vi "Test Billete 100.vi"(8 "error in (no error)":errorcluster, 11 "TestCase in":refnum<class "Unit Test Proy.lvclass">) -> (0 "error out":errorcluster, 3 "TestCase out":refnum<class "Unit Test Proy.lvclass">)   [LabVIEW 2020, in "Unit Test Proy.lvclass"]
uses:
  Unit Test Proy.lvclass
  Dinero/Dinero.lvclass
  Dinero/Dinero.lvclass/Dinero.ctl
  <vilib>/addons/_JKI Toolkits/VI Tester/TestCase.llb/TestCase.lvclass
  C:/Program Files (x86)/National Instruments/LabVIEW 2020/vi.lib/addons/_JKI Toolkits/VI Tester/TestCase.llb/TestCase.lvclass
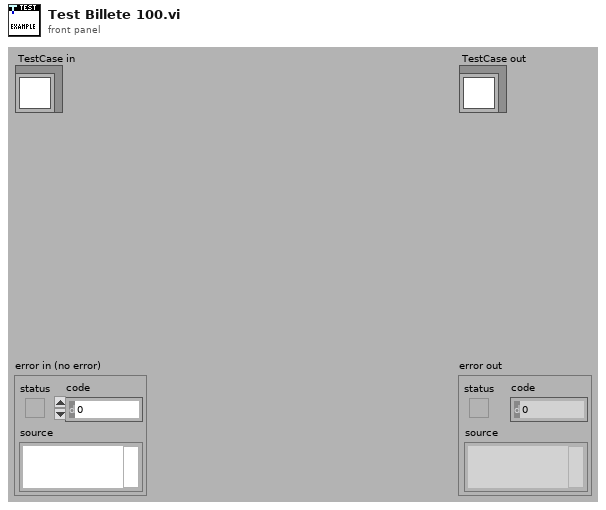
[diagram p1: front panel]
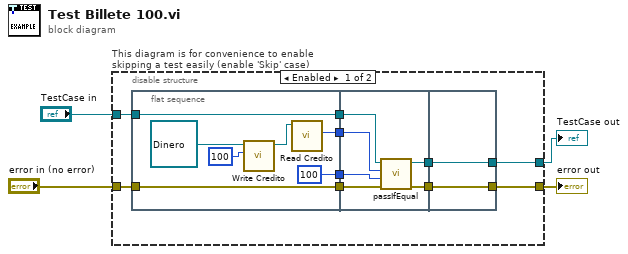
[diagram p0: block diagram]
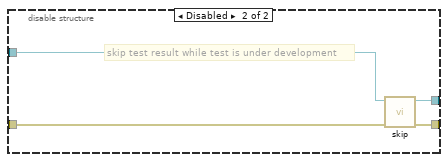
[diagram p2: hidden frame]
diagram:
  n1 = disable-structure "This diagram is for convenience to enable skipping a test easily (enable 'Skip' case)" shown="Enabled" {
    disable-tunnel: "TestCase in" -> [w7 w33]
    disable-tunnel: [w12 w31] -> w1
    disable-tunnel: [w11 w32] -> w3
    disable-tunnel: "error in (no error)" -> [w14 w30]
    frame Enabled {
      n2 = flat-sequence {
        tunnel: w14 -> [w21]
        tunnel: [w21] -> w9
        tunnel: [w20] -> w8
        tunnel: w7 -> [w20]
        tunnel: [w17] -> w6
        tunnel: [100] -> w5
        tunnel: [w27] -> w13
        tunnel: [w26] -> w10
        tunnel: w9 -> [w25]
        tunnel: w8 -> [w24]
        tunnel: w6 -> [w23]
        tunnel: w5 -> [w22]
        tunnel: w13 -> [w29]
        tunnel: [w29] -> w12
        tunnel: [w28] -> w11
        tunnel: w10 -> [w28]
        frame #0 {
          n3 = call "Write Credito.vi"("Credito"=100, "Dinero in"=refnum<class "Dinero.lvclass"> refnum ("Dinero.lvlib:Dinero.lvclass")) -> ("Dinero out"=w18:refnum<class "Dinero.lvclass">)  [unwired: 8 in, 1 out]
          n4 = call "Read Credito.vi"("Dinero in"=w18) -> ("Credito"=w17:i32)  [unwired: 8 in, 2 out]
        }
        frame #1 {
          n5 = call-dynamic "passIfEqual.vi"("error in (no error)"=w25, "y"=w22, "x"=w23, "TestCase in"=w24) -> ("error out"=w26:errorcluster, "TestCase out"=w27:refnum<class "Unit Test Proy.lvclass">)  [unwired: 6 in]
        }
        frame #2 {
        }
      }
    }
    frame Disabled {
      # "skip test result while test is under development"
      n6 = call <vilib>:"skip.vi"("error in (no error)"=w30, "TestCase in"=w33) -> ("error out"=w32:errorcluster, "TestCase out"=w31:refnum<class "Unit Test Proy.lvclass">)  [unwired: 8 in]
    }
  }
  "error out" <- w3
  "TestCase out" <- w1
